vi "Read Logic Datas Trigger Point.vi"() -> (3 "function return":u32)   [LabVIEW 2021, in "vmmso.lvlib"]
doc: "DLL_API unsigned int WINAPI ReadLogicDatasTriggerPoint();"
uses:
  vmmso.lvlib
  vmmso.dll
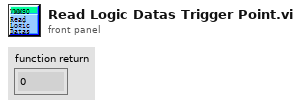
[diagram p1: front panel]
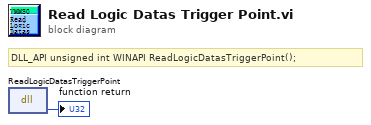
[diagram p0: block diagram]
diagram:
  # "DLL_API unsigned int WINAPI ReadLogicDatasTriggerPoint();"
  n1 = dll-call lib="D:/labviewdemo/LabviewDemo 21/vmmso/vmmso.*" fn="ReadLogicDatasTriggerPoint"() -> (→"function return":u32)  [unwired: 3 in, 2 out]
